vi "CohortCheck.vi"(11 "Cohort.lvclass":refnum<class "Cohort.lvclass">) -> (0 "error out":errorcluster)   [LabVIEW 2012, in "Cohort.lvclass"]
uses:
  Cohort.lvclass
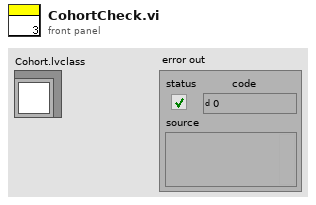
[diagram p1: front panel]
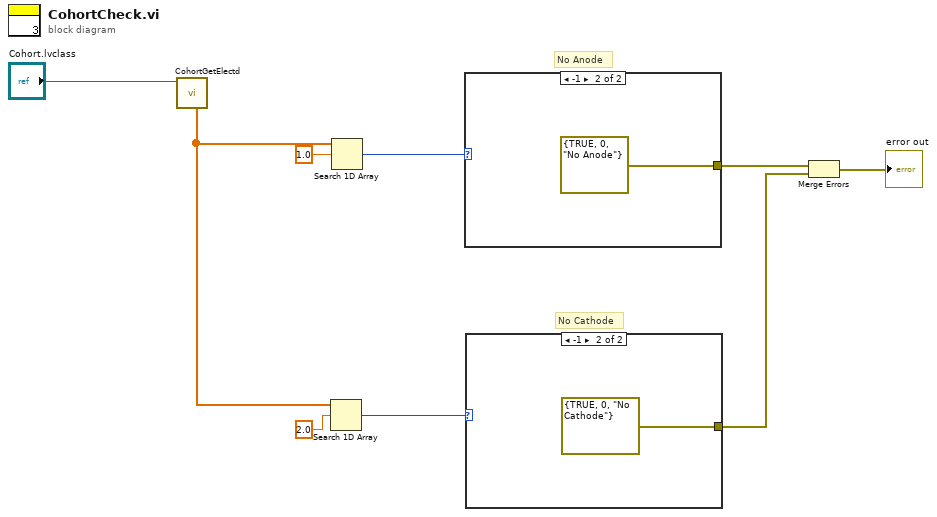
[diagram p0: block diagram]
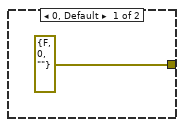
[diagram p2: hidden frame]
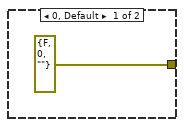
[diagram p3: hidden frame]
diagram:
  # "No Cathode"
  # "No Anode"
  n1 = call-dynamic "CohortGetElectd.vi"("Cohort in"="Cohort.lvclass") -> ("Amplitude"=w6:sgl[])  [unwired: 7 in, 3 out]
  n2 = Search 1D Array(1D array=w6, element=sgl 2.0) -> (index of element=w3:i32)  [unwired: 1 in]
  n3 = Search 1D Array(1D array=w6, element=sgl 1.0) -> (index of element=w5:i32)  [unwired: 1 in]
  n4 = case shown="-1" w5 {
    tunnel: [errorcluster {"status"=FALSE, "code"=0, "source"=""} ("error constant") errorcluster {TRUE, 0, "No Anode"}] -> w4
    frame 0, Default {
    }
    frame -1 {
    }
  }
  n5 = case shown="-1" w3 {
    tunnel: [errorcluster {"status"=FALSE, "code"=0, "source"=""} ("error constant") errorcluster {TRUE, 0, "No Cathode"}] -> w2
    frame 0, Default {
    }
    frame -1 {
    }
  }
  n6 = Merge Errors(w4, w2) -> (→"error out":errorcluster)
